vi "Operate Grabber.vi"(8 "error in (no error)":errorcluster, 10 "Joystick State":T1, 11 "Operator in":refnum<class "Operator.lvclass">) -> (0 "error out":errorcluster, 3 "Operator out":refnum<class "Operator.lvclass">)   [LabVIEW 2014, in "Operator.lvlib" / "Operator.lvclass"]
uses:
  Operator.lvclass
  Joystick/Joystick Class/Joystick State.ctl
  Joystick/Joystick Class/Button State.ctl
  Joystick/Joystick Class/Axis State.ctl
  Operator.lvclass/Operator.ctl
  Grabber/Grabber Messages/Spin Wheels Msg/Spin Wheels Msg.lvclass/Spin Wheels Msg.ctl
  <vilib>/ActorFramework/Message Enqueuer/Message Enqueuer.lvclass/Message Enqueuer.ctl
  <vilib>/ActorFramework/Message Enqueuer/Enqueue.vi
  <vilib>/ActorFramework/Message Priority Queue/Priority Enqueue.vi
  Grabber/Grabber Messages/Spin Wheels Msg/Spin Wheels Msg.lvclass
  Grabber/Grabber Messages/Close Arms Msg/Close Arms Msg.lvclass
  Grabber/Grabber Messages/Open Arms Msg/Open Arms Msg.lvclass
  Joystick/Joystick Class/Joystick.lvclass
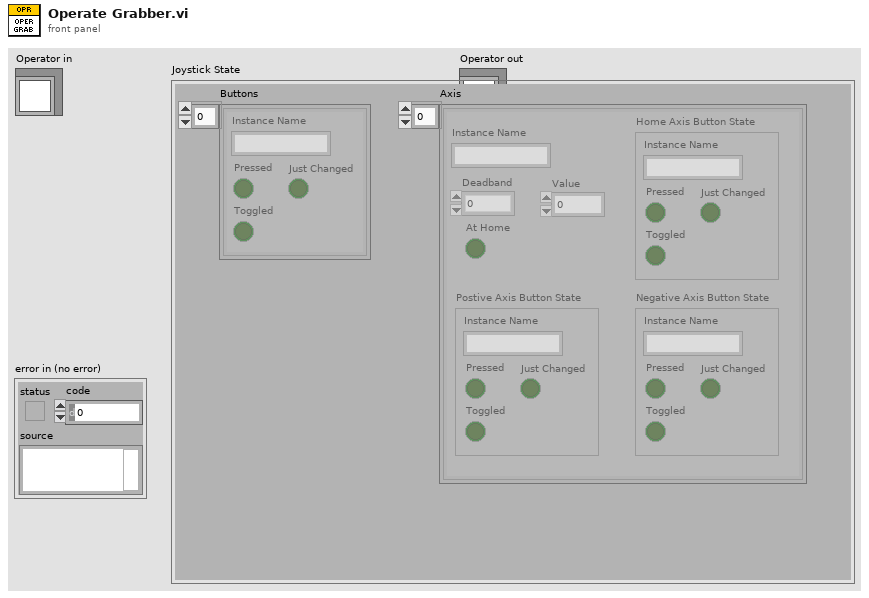
[diagram p1: front panel]
types:
  T1 = typedef "Joystick.lvlib/Joystick.lvclass/Joystick State.ctl" = cluster{"Buttons":T2[], "Axis":T3[]}
  T2 = typedef "Joystick.lvlib/Joystick.lvclass/Button State.ctl" = cluster{"Pressed":bool, "Instance Name":string, "Toggled":bool, "Just Changed":bool}
  T3 = typedef "Joystick.lvlib/Joystick.lvclass/Axis State.ctl" = cluster{"Instance Name":string, "Deadband":dbl, "Value":dbl, "At Home":bool, "Postive Axis Button State":T2, "Negative Axis Button State":T2, "Home Axis Button State":T2}
  T4 = enum16{"Critical", "Error", "Warning", "Informational", "Debug"}
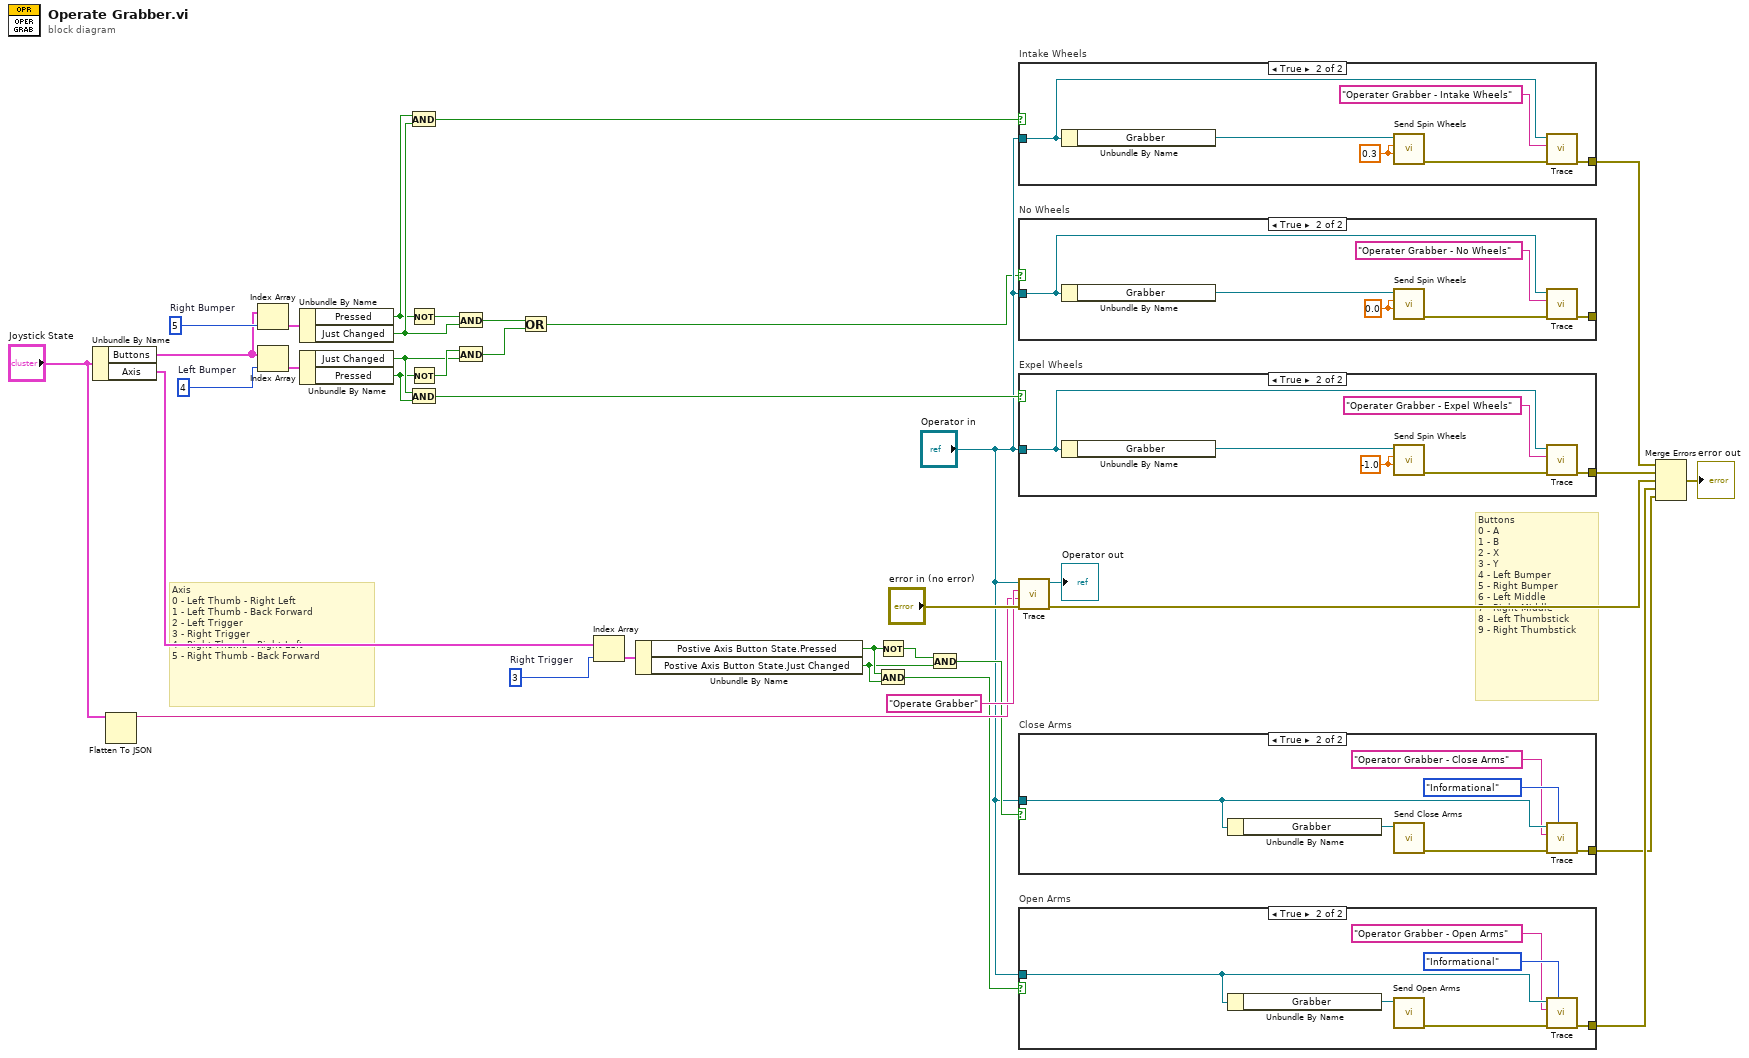
[diagram p0: block diagram]
diagram:
  w25 = 3  # Right Trigger
  w28 = 5  # Right Bumper
  w30 = 4  # Left Bumper
  # "Buttons\n0 - A\n1 - B\n2 - X\n3 - Y\n4 - Left Bumper\n5 - Right Bumper\n6 - Left Middle\n7 - Right Middle\n8 - Left Thumbstick\n9 - Right Thumbstick"
  # "Axis\n0 - Left Thumb - Right Left\n1 - Left Thumb - Back Forward\n2 - Left Trigger\n3 - Right Trigger\n4 - Right Thumb - Right Left\n5 - Right Thumb - Back Forward"
  n1 = Unbundle By Name("Joystick State") -> ("Buttons"=w27:T2[], "Axis"=w26:T3[])
  n2 = Flatten To JSON(anything="Joystick State") -> (JSON string=w32:string)  [unwired: 2 in, 1 out]
  n3 = Index Array(array=w27, index=w28) -> (element=w12:T2)
  n4 = Index Array(array=w27, index=w30) -> (element=w29:T2)
  n5 = Unbundle By Name(w12) -> ("Pressed"=w6:bool, "Just Changed"=w8:bool)
  n6 = Unbundle By Name(w29) -> ("Just Changed"=w4:bool, "Pressed"=w1:bool)
  n7 = And(x=w6, y=w8) -> (x .and. y?=w11:bool)
  n8 = Not(x=w6) -> (.not. x?=w9:bool)
  n9 = Not(x=w1) -> (.not. x?=w5:bool)
  n10 = And(x=w4, y=w1) -> (x .and. y?=w15:bool)
  n11 = And(x=w9, y=w8) -> (x .and. y?=w7:bool)
  n12 = And(x=w5, y=w4) -> (x .and. y?=w3:bool)
  n13 = Or(x=w7, y=w3) -> (x .or. y?=w2:bool)
  n14 = Index Array(array=w26, index=w25) -> (element=w24:T3)
  n15 = Unbundle By Name(w24) -> ("Postive Axis Button State.Pressed"=w23:bool, "Postive Axis Button State.Just Changed"=w21:bool)
  n16 = Not(x=w23) -> (.not. x?=w22:bool)
  n17 = And(x=w23, y=w21) -> (x .and. y?=w17:bool)
  n18 = And(x=w22, y=w21) -> (x .and. y?=w16:bool)
  n19 = case "Intake Wheels" shown="True" w11 {
    tunnel: "Operator in" -> [_ w39]
    tunnel: [_ w37] -> w13
    frame False {
    }
    frame True {
      w42 = 0.3 ("Left Wheel Power")
      n20 = Unbundle By Name(w39) -> ("Grabber"=w41:refnum<class "Message Enqueuer.lvclass">)
      n21 = call "Send Spin Wheels.vi"("Right Wheel Power"=w42, "Left Wheel Power"=w42, "Message Enqueuer"=w41) -> ("error out"=w40:errorcluster)  [unwired: 7 in, 1 out]
      n22 = call-dynamic "Trace.vi"("error in (no error)"=w40, "System Action"="Operater Grabber - Intake Wheels", "System Actor in"=w39) -> ("error out"=w37:errorcluster)  [unwired: 7 in, 1 out]
    }
  }
  n23 = case "No Wheels" shown="True" w2 {
    tunnel: "Operator in" -> [_ w45]
    tunnel: [_ w43] -> _
    frame False {
    }
    frame True {
      w48 = 0.0 ("Left Wheel Power")
      n24 = Unbundle By Name(w45) -> ("Grabber"=w47:refnum<class "Message Enqueuer.lvclass">)
      n25 = call "Send Spin Wheels.vi"("Right Wheel Power"=w48, "Left Wheel Power"=w48, "Message Enqueuer"=w47) -> ("error out"=w46:errorcluster)  [unwired: 7 in, 1 out]
      n26 = call-dynamic "Trace.vi"("error in (no error)"=w46, "System Action"="Operater Grabber - No Wheels", "System Actor in"=w45) -> ("error out"=w43:errorcluster)  [unwired: 7 in, 1 out]
    }
  }
  n27 = case "Expel Wheels" shown="True" w15 {
    tunnel: "Operator in" -> [_ w51]
    tunnel: [_ w49] -> w14
    frame False {
    }
    frame True {
      w54 = -1.0 ("Left Wheel Power")
      n28 = Unbundle By Name(w51) -> ("Grabber"=w53:refnum<class "Message Enqueuer.lvclass">)
      n29 = call "Send Spin Wheels.vi"("Right Wheel Power"=w54, "Left Wheel Power"=w54, "Message Enqueuer"=w53) -> ("error out"=w52:errorcluster)  [unwired: 7 in, 1 out]
      n30 = call-dynamic "Trace.vi"("error in (no error)"=w52, "System Action"="Operater Grabber - Expel Wheels", "System Actor in"=w51) -> ("error out"=w49:errorcluster)  [unwired: 7 in, 1 out]
    }
  }
  n31 = call-dynamic "Trace.vi"("error in (no error)"="error in (no error)", "System Message"=w32, "System Action"="Operate Grabber", "System Actor in"="Operator in") -> ("error out"=w34:errorcluster, "System Actor out"=→"Operator out":refnum<class "Operator.lvclass">)  [unwired: 6 in]
  n32 = case "Close Arms" shown="True" w16 {
    tunnel: "Operator in" -> [_ w58]
    tunnel: [_ w55] -> w18
    frame False {
    }
    frame True {
      n33 = Unbundle By Name(w58) -> ("Grabber"=w60:refnum<class "Message Enqueuer.lvclass">)
      n34 = call "Send Close Arms.vi"("Message Enqueuer"=w60) -> ("error out"=w59:errorcluster)  [unwired: 9 in, 1 out]
      n35 = call-dynamic "Trace.vi"("Trace Level"=T4."Informational", "error in (no error)"=w59, "System Action"="Operator Grabber - Close Arms", "System Actor in"=w58) -> ("error out"=w55:errorcluster)  [unwired: 6 in, 1 out]
    }
  }
  n36 = case "Open Arms" shown="True" w17 {
    tunnel: "Operator in" -> [_ w66]
    tunnel: [_ w61] -> w19
    frame False {
    }
    frame True {
      n37 = Unbundle By Name(w66) -> ("Grabber"=w63:refnum<class "Message Enqueuer.lvclass">)
      n38 = call "Send Open Arms.vi"("Message Enqueuer"=w63) -> ("error out"=w62:errorcluster)  [unwired: 9 in, 1 out]
      n39 = call-dynamic "Trace.vi"("Trace Level"=T4."Informational", "error in (no error)"=w62, "System Action"="Operator Grabber - Open Arms", "System Actor in"=w66) -> ("error out"=w61:errorcluster)  [unwired: 6 in, 1 out]
    }
  }
  n40 = Merge Errors(w13, w14, w34, w19, w18) -> (→"error out":errorcluster)
